vi "Read Camera.vi"(8 "error in (no error)":errorcluster, 10 "Camera Name":string, 11 "Gantry Class in":refnum<class "Gantry.lvclass">) -> (0 "error out":errorcluster, 2 "Camera":T1, 3 "Gantry Class out":refnum<class "Gantry.lvclass">)   [LabVIEW 2022 SP3, in "Gantry.lvclass"]
uses:
  Gantry.lvclass
  External/Vision/camera.ctl
  External/Vision/camera driver.ctl
  Gantry.lvclass/Gantry.ctl
  External/Vision/Vision.lvlib
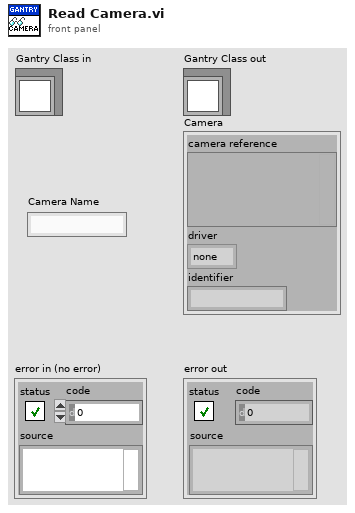
[diagram p1: front panel]
types:
  T1 = typedef "Vision.lvlib/camera.ctl" = cluster{"camera reference":variant, "driver":T2, "identifier":string}
  T2 = typedef "Vision.lvlib/camera driver.ctl" = enum16{"none", "ueye", "wmf"}
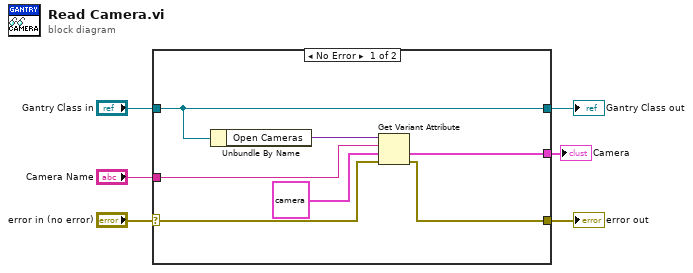
[diagram p0: block diagram]
diagram:
  n1 = case shown="No Error" "error in (no error)" {
    selector: "error in (no error)" -> [w10 w15]
    tunnel: [w8 w15] -> w5
    tunnel: [w13 w14] -> w3
    tunnel: "Gantry Class in" -> [w13 w14]
    tunnel: "Camera Name" -> [w11 _]
    tunnel: [w9 _] -> w1
    frame No Error {
      n2 = Unbundle By Name(w13) -> ("Open Cameras"=w12:variant)
      n3 = Get Variant Attribute(Variant=w12, name=w11, default value (empty Variant)=T1 {"camera reference"=variant, "driver"=enum."none", "identifier"=""} ("Cluster"), error in=w10) -> (value=w9:T1, error out=w8:errorcluster)  [unwired: 2 out]
    }
    frame Error {
    }
  }
  "error out" <- w5
  "Gantry Class out" <- w3
  "Camera" <- w1
